vi "SubSystems.vi"(8 "error in":errorcluster) -> ()   [LabVIEW 2018]
doc: "This VI calls the various robot subsystems that will then run in parallel. New subSystems will automatlically script code to make the call."
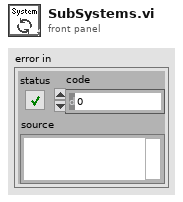
[diagram p1: front panel]
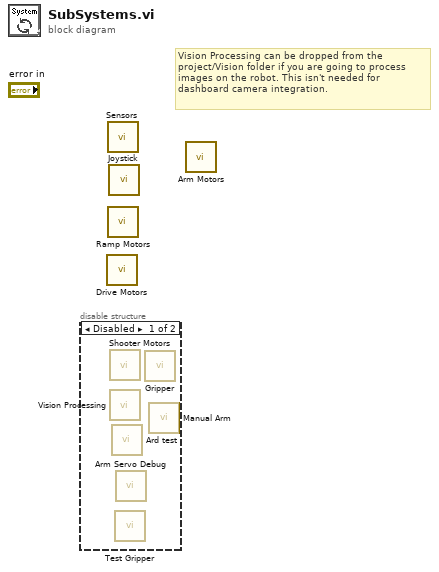
[diagram p0: block diagram]
diagram:
  # "Vision Processing can be dropped from the\nproject/Vision folder if you are going to process\nimages on the robot. This isn't needed for\ndashboard camera integration."
  n1 = disable-structure shown="Disabled" {
    frame Disabled {
      n2 = call "Shooter Motors.vi"() -> ()  [unwired: 12 in]
      n3 = call "Vision Processing.vi"() -> ()  [unwired: 8 in]
      n4 = call "Ard test.vi"() -> ()  [unwired: 12 in]
      n5 = call "Test Gripper.vi"() -> ()  [unwired: 12 in]
      n6 = call "Arm Servo Debug.vi"() -> ()  [unwired: 12 in]
      n7 = call "Gripper.vi"() -> ()  [unwired: 12 in]
      n8 = call "Manual Arm.vi"() -> ()  [unwired: 12 in]
    }
    frame Enabled {
    }
  }
  n9 = call "Drive Motors.vi"() -> ()  [unwired: 12 in]
  n10 = call "Sensors.vi"() -> ()  [unwired: 12 in]
  n11 = call "Ramp Motors.vi"() -> ()  [unwired: 12 in]
  n12 = call "Joystick.vi"() -> ()  [unwired: 12 in]
  n13 = call "Arm Motors.vi"() -> ()  [unwired: 12 in]
